vi "Write Symbol.vi"(6 "Data":variant, 8 "Error In":errorcluster, 10 "Symbol Name":string, 11 "AMS Connection":T1) -> (0 "Error Out":errorcluster, 3 "Success":bool)   [LabVIEW 2020, in "TwinCAT ADS.lvlib" / "PLC.lvlib"]
doc: "Write the symbol with <b>Symbol Name</b>. <b>Data</b> is a variant, accepting any LabVIEW data type although some may not be supported by the internal conversion.\n\nStrings are only supported with a fix length of 80 characters."
uses:
  <userlib>/PMA/High Level/PLC/PLC.lvlib
  <userlib>/PMA/Low Level/TypeDefs/AMS Connection.ctl
  <userlib>/PMA/Low Level/TypeDefs/AMS.ctl
  <userlib>/PMA/TwinCAT ADS.lvlib
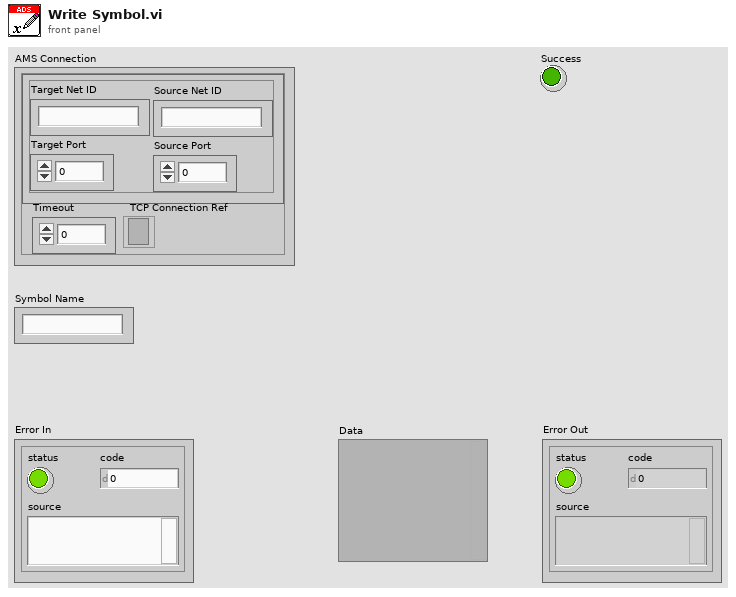
[diagram p1: front panel]
types:
  T1 = typedef "TwinCAT ADS.lvlib/AMS Connection.ctl" = cluster{"AMS":T2, "Timeout":i32, "TCP Connection Ref":refnum<k5>}
  T2 = typedef "TwinCAT ADS.lvlib/AMS.ctl" = cluster{"Target Net ID":string, "Target Port":u16, "Source Net ID":string, "Source Port":u16}
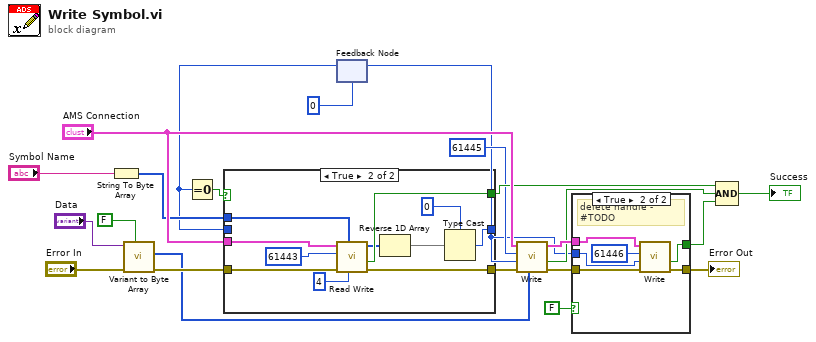
[diagram p0: block diagram]
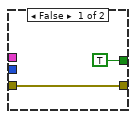
[diagram p2: hidden frame]
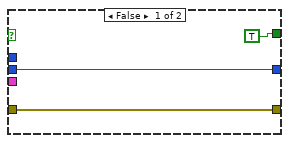
[diagram p3: hidden frame]
diagram:
  n1 = String To Byte Array(string="Symbol Name") -> (unsigned byte array=w15:u8[])
  n2 = call <userlib>:"Variant to Byte Array.vi"("InStruct"=FALSE ("RISC"), "Error In"="Error In", "Variant"="Data") -> ("Error Out"=w6:errorcluster, "Byte Stream Out"=w5:u8[])  [unwired: 7 in]
  n3 = feedback #1(u32 0) -> (w2:u32)
  n4 = Equal To 0?(x=w2) -> (x = 0?=w3:bool)
  n5 = case shown="True" w3 {
    tunnel: "AMS Connection" -> [_ w36]
    tunnel: [w23 w35] -> w17
    tunnel: w15 -> [_ w34]
    tunnel: [TRUE ("Success") w33] -> w13
    tunnel: [w25 w32] -> w9
    tunnel: w2 -> [w25 _]
    tunnel: w6 -> [w23 w26]
    frame False {
    }
    frame True {
      n6 = call <userlib>:"Read Write.vi"("Read Length"=u32 4, "Write Data"=w34, "Error In"=w26, "Index Group"=u32 61443, "AMS Connection In"=w36) -> ("Error Out"=w35:errorcluster, "Success"=w33:bool, "Read Data"=w30:u8[])  [unwired: 3 in, 1 out]
      n7 = Reverse 1D Array(array=w30) -> (reversed array=w31:u8[])
      n8 = Type Cast(type=u32 0, x=w31) -> (*(type *) &x=w32:u32)
    }
  }
  n9 = feedback-in #1(w9) -> ()
  n10 = call <userlib>:"Write.vi"("Data"=w5, "Error In"=w17, "Offset"=w9, "Index Group"=u32 61445, "AMS Connection In"="AMS Connection") -> ("Error Out"=w16:errorcluster, "Success"=w11:bool, "AMS Connection Out"=w18:T1)  [unwired: 3 in, 1 out]
  n11 = case shown="True" FALSE {
    tunnel: [w37 w44] -> w19
    tunnel: w18 -> [_ w43]
    tunnel: w16 -> [w37 w42]
    tunnel: [TRUE ("Success") w40] -> w12
    tunnel: w9 -> [_ w39]
    frame False {
    }
    frame True {
      # "delete handle - #TODO"
      n12 = call <userlib>:"Write.vi"("Error In"=w42, "Offset"=w39, "Index Group"=u32 61446, "AMS Connection In"=w43) -> ("Error Out"=w44:errorcluster, "Success"=w40:bool)  [unwired: 4 in, 2 out]
    }
  }
  "Error Out" <- w19
  n13 = Compound Arithmetic op=AND(w13, w11, w12) -> (→"Success":bool)
